vi "R5NaSignalProcess.vi"(9 "error":errorcluster, 11 "LabVIEW Web Service":refnum<class "Web Service.lvclass">) -> (1 "error out":errorcluster)   [LabVIEW 2016]
uses:
  <vilib>/wsapi/Web Service.lvclass
  Controls/Tri State Control.ctl
  Controls/ISE.ctl
panel:
  out "R1Na":T1 {"Steady State?" items=["False", "True", "NaN", ""]}
  out "output array":dbl[][](array[numeric])
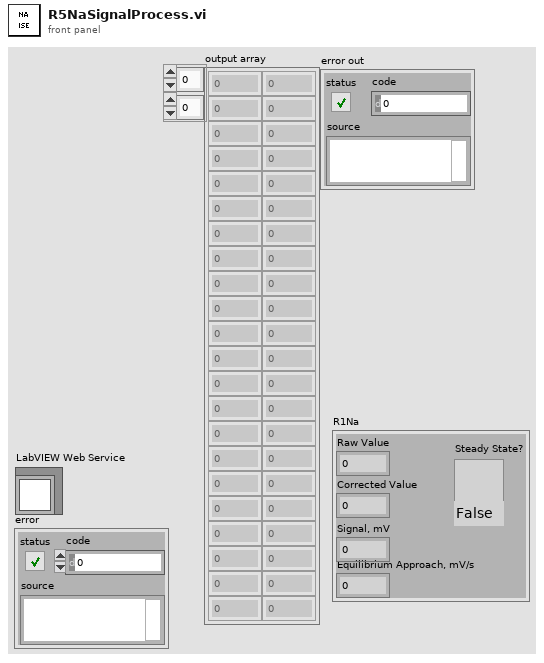
[diagram p1: front panel]
types:
  T1 = typedef "ISE.ctl" = cluster{"Raw Value":dbl, "Corrected Value":dbl, "Signal, mV":dbl, "Equilibrium Approach, mV/s":dbl, "Steady State?":T2}
  T2 = typedef "Tri State Control.ctl" = u16
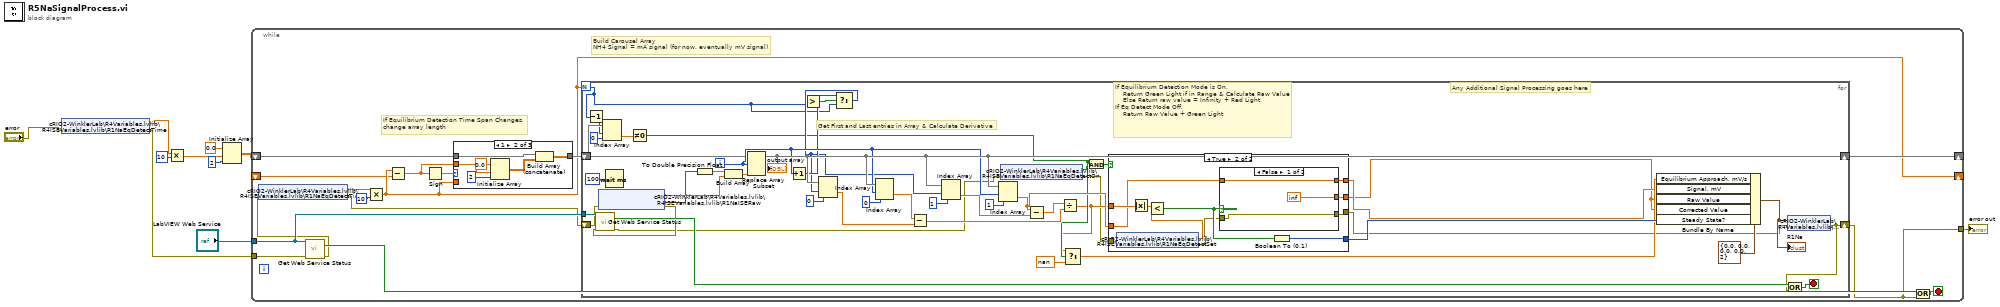
[diagram p0: block diagram]
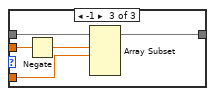
[diagram p3: hidden frame]
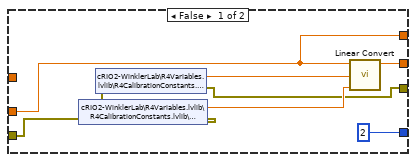
[diagram p4: hidden frame]
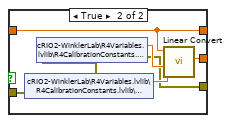
[diagram p5: hidden frame]
diagram:
  n1 = shared-variable "cRIO2-WinklerLab\\R4Variables.lvlib\\R4ISEVariables.lvlib\\R1NaEqDetectTime"(error in="error") -> (w3:dbl, error out=w2:errorcluster)
  n2 = Multiply(x=w3, y=10) -> (x*y=w5:dbl)
  n3 = Initialize Array(0.0 ("element"), w5, 2 ("dimension size")) -> (w6:dbl[][])
  n4 = while {
    tunnel: "LabVIEW Web Service" -> [w26]
    tunnel: w2 -> [w16]
    shift-right: [w20] -> _
    shift-left: w6 -> [w23]
    shift-right: [w19] -> _
    shift-left: _ -> [w18]
    tunnel: [w11] -> w1
    stop <- w15 stop-if-true
    # "Build Carousel Array\nNH4 Signal = mA signal (for now, eventually mV signal)"
    # "If Equilibrium Detection Time Span Changes, \nchange array length"
    n5 = call <vilib>:"Get Web Service Status.vi"("LabVIEW Web Service"=w26, "error in (no error)"=w16) -> ("service stopping?"=w17:bool, "error out"=w14:errorcluster)  [unwired: 11 in, 1 out]
    n6 = shared-variable "cRIO2-WinklerLab\\R4Variables.lvlib\\R4ISEVariables.lvlib\\R1NaEqDetectTime"(error in=w14) -> (w13:dbl, error out=w12:errorcluster)
    n7 = Multiply(x=w13, y=10) -> (x*y=w19:dbl)
    n8 = Subtract(x=w19, y=w18) -> (x-y=w22:dbl)
    n9 = Sign(1:w22) -> (0:w24:dbl)
    n10 = case shown="1" w24 {
      tunnel: w23 -> [w27 w31 w34]
      tunnel: w22 -> [_ w28 w36]
      tunnel: [w27 w29 w38] -> w21
      tunnel: w19 -> [_ _ w37]
      frame 0, Default {
      }
      frame 1 {
        n11 = Initialize Array(0.0 ("element"), w28, 2 ("dimension size")) -> (w30:dbl[][])
        n12 = Build Array (concatenate)(w31, w30) -> (w29:dbl[][])
      }
      frame -1 {
        n13 = Negate(x=w36) -> (-x=w35:dbl)
        n14 = Array Subset(array=w34, index (row)=w35, length (row)=w37) -> (w38:dbl[][])  [unwired: 2 in]
      }
    }
    n15 = for {
      N: w19 -> [w53]
      tunnel: w26 -> [w83]
      shift-right: [w71] -> w20
      shift-left: w21 -> [w64]
      shift-right: [w41] -> w11
      shift-left: w12 -> [w46]
      i -> [w70]
      stop <- w50 stop-if-true
      # "Any Additional Signal Processing goes here"
      # "If Equilibrium Detection Mode is On, \n    Return Green Light if in Range & Calculate Raw Value\n    Else Return raw value = Infinity + Red Light\nIf Eq Detect Mode Off,\n    Return Raw Value + Green Light"
      # "Get First and Last entries in Array & Calculate Derivative"
      n16 = Decrement(x=w53) -> (x-1=w54:i32)
      n17 = shared-variable "cRIO2-WinklerLab\\R4Variables.lvlib\\R4ISEVariables.lvlib\\R1NaISERaw"(error in=w46) -> (w49:dbl, error out=w47:errorcluster, w48:timestamp)
      n18 = call <vilib>:"Get Web Service Status.vi"("LabVIEW Web Service"=w83, "error in (no error)"=w47) -> ("service stopping?"=w51:bool, "error out"=w45:errorcluster)  [unwired: 11 in, 1 out]
      n19 = Index Array(array=w64, index (row)=w54, index (col)=0 ("disabled index (col)")) -> (element=w62:dbl)
      n20 = Wait (ms)(milliseconds to wait=u32 100) -> ()  [unwired: 1 out]
      n21 = Not Equal To 0?(x=w62) -> (x != 0?=w59:bool)
      n22 = To Double Precision Float(number=w48) -> (double precision float=w82:dbl)
      n23 = Build Array(w82, w49) -> (w81:dbl[])
      n24 = Replace Array Subset(array=w64, new element=w81, index (row)=w70) -> (w71:dbl[][])  [unwired: 1 in]
      "output array" <- w71
      n25 = Increment(x=w70) -> (x+1=w66:i32)
      n26 = Greater?(x=w66, y=w53) -> (0:w67:bool)
      n27 = Select(t=w66, s=w67, f=w53) -> (s? t:f=w65:i32)
      n28 = Index Array(array=w71, index (row)=w65, index (col)=0 ("disabled index (col)")) -> (element=w73:dbl)
      n29 = Index Array(array=w71, index (row)=w70, index (col)=0 ("disabled index (col)")) -> (element=w68:dbl)
      n30 = Subtract(x=w68, y=w73) -> (x-y=w79:dbl)
      n31 = Index Array(array=w71, index (row)=w65, index (col)=1 ("disabled index (col)")) -> (element=w72:dbl)
      n32 = Index Array(array=w71, index (row)=w70, index (col)=1 ("disabled index (col)")) -> (element=w60:dbl)
      n33 = shared-variable "cRIO2-WinklerLab\\R4Variables.lvlib\\R4ISEVariables.lvlib\\R1NaEqDetectOn"(error in=w45) -> (w39:bool, error out=w44:errorcluster)
      n34 = Subtract(x=w60, y=w72) -> (x-y=w78:dbl)
      n35 = Divide(x=w78, y=w79) -> (x/y=w57:dbl)
      n36 = Select(t=w57, s=w59, f=nan) -> (s? t:f=w56:dbl)
      n37 = And(x=w59, y=w39) -> (x .and. y?=w61:bool)
      n38 = case shown="True" w61 {
        tunnel: [w87 w102] -> w43
        tunnel: [w90 w101] -> w55
        tunnel: w57 -> [_ w100]
        tunnel: [2 w98] -> w69
        tunnel: w60 -> [w90 w97]
        tunnel: w44 -> [w86 w93]
        tunnel: [w84 w95] -> w40
        frame False {
          n39 = shared-variable "cRIO2-WinklerLab\\R4Variables.lvlib\\R4CalibrationConstants.lvlib\\R4NH4Intercept"(error in=w86) -> (w89:dbl, error out=w85:errorcluster)
          n40 = shared-variable "cRIO2-WinklerLab\\R4Variables.lvlib\\R4CalibrationConstants.lvlib\\R4NH4Slope"(error in=w85) -> (w88:dbl, error out=w84:errorcluster)
          n41 = call "Linear Convert.vi"("Intercept"=w89, "Slope"=w88, "Signal"=w90) -> ("Result"=w87:dbl)  [unwired: 8 in]
        }
        frame True {
          n42 = shared-variable "cRIO2-WinklerLab\\R4Variables.lvlib\\R4ISEVariables.lvlib\\R1NaEqDetectSet"(error in=w93) -> (w94:dbl, error out=w92:errorcluster)
          n43 = Absolute Value(x=w100) -> (abs(x)=w96:dbl)
          n44 = Less?(x=w96, y=w94) -> (x < y?=w99:bool)
          n45 = case shown="False" w99 {
            tunnel: [inf w111] -> w102
            tunnel: [w104 w112] -> w101
            tunnel: w97 -> [w104 w112]
            tunnel: w92 -> [w103 w108]
            tunnel: [w103 w106] -> w95
            frame False {
            }
            frame True {
              n46 = shared-variable "cRIO2-WinklerLab\\R4Variables.lvlib\\R4CalibrationConstants.lvlib\\R4NH4Intercept"(error in=w108) -> (w110:dbl, error out=w107:errorcluster)
              n47 = shared-variable "cRIO2-WinklerLab\\R4Variables.lvlib\\R4CalibrationConstants.lvlib\\R4NH4Slope"(error in=w107) -> (w109:dbl, error out=w106:errorcluster)
              n48 = call "Linear Convert.vi"("Intercept"=w110, "Slope"=w109, "Signal"=w112) -> ("Result"=w111:dbl)  [unwired: 8 in]
            }
          }
          n49 = Boolean To (0,1)(Boolean=w99) -> (0, 1=w98:i16)
        }
      }
      n50 = Bundle By Name(cluster=T1 {"Raw Value"=0.0, "Corrected Value"=0.0, "Signal, mV"=0.0, "Equilibrium Approach, mV/s"=0.0, "Steady State?"=2} ("R1NH4"), "Equilibrium Approach, mV/s"=w56, "Signal, mV"=w55, "Raw Value"=w43, "Corrected Value"=w43, "Steady State?"=w69) -> (w42:T1)
      "R1Na" <- w42
      n51 = shared-variable "cRIO2-WinklerLab\\R4Variables.lvlib\\R4Signals.lvlib\\R1Na"(w42, error in=w40) -> (error out=w41:errorcluster)
      n52 = Or(x=w51, y=w41) -> (x .or. y?=w50:bool)
    }
    n53 = Or(x=w17, y=w11) -> (x .or. y?=w15:bool)
  }
  "error out" <- w1
